vi "hardware_initialize_hardware.vi"(8 "error in (no error)":errorcluster, 11 "thorlabs_kinesis in":refnum<class "thorlabs_kinesis.lvclass">) -> (0 "error out":errorcluster, 3 "thorlabs_kinesis out":refnum<class "thorlabs_kinesis.lvclass">)   [LabVIEW 2015, in "thorlabs_kinesis.lvclass"]
uses:
  thorlabs_kinesis.lvclass
  thorlabs_kinesis.lvclass/thorlabs_kinesis.ctl
  thorlabs_drivers/Thorlabs.MotionControl.Benchtop.Piezo.dll
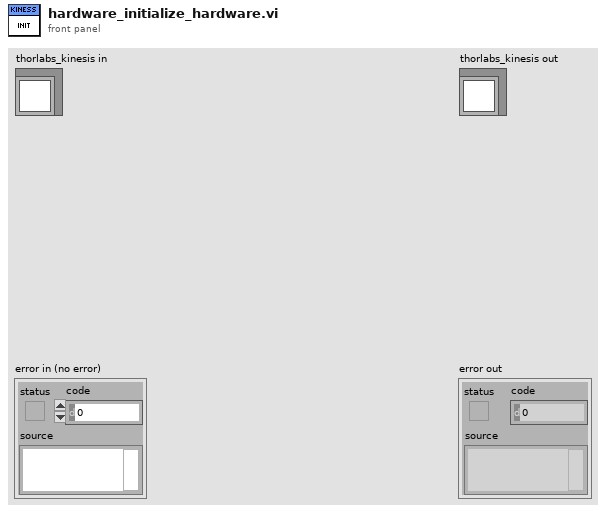
[diagram p1: front panel]
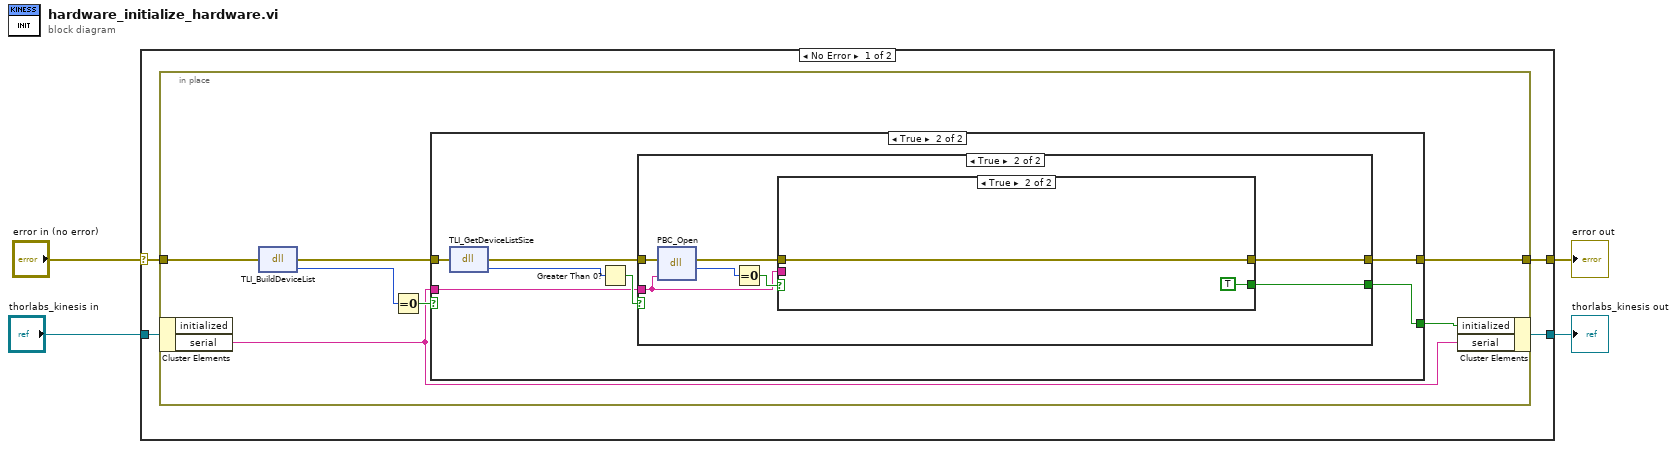
[diagram p0: block diagram]
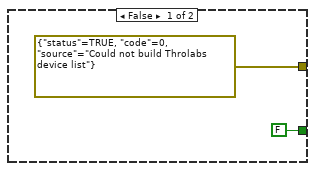
[diagram p2: hidden frame]
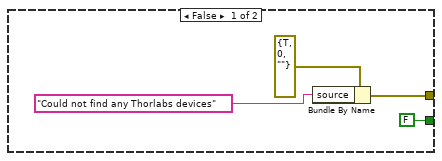
[diagram p3: hidden frame]
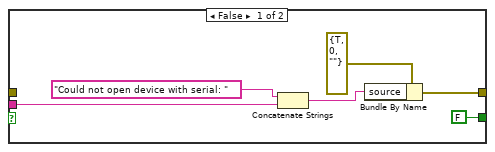
[diagram p4: hidden frame]
diagram:
  n1 = case shown="No Error" "error in (no error)" {
    selector: "error in (no error)" -> [w7 w44]
    tunnel: "thorlabs_kinesis in" -> [w8 w45]
    tunnel: [w6 w44] -> w2
    tunnel: [w5 w45] -> w1
    frame No Error {
      n2 = in-place {
        in-place-border: w7 -> [w15]
        in-place-border: [w10] -> w6
        n3 = in-place-cluster #1(w8) -> ("serial"=w11:string)  [unwired: 1 out]
        n4 = dll-call lib="C:/Users/bspoka/Documents/LabVIEW Data/lview_180307/Stage Class/Thorlabs Kinesis/thorlabs_drivers/Thorlabs.MotionControl.Benchtop.Piezo.dll" fn="TLI_BuildDeviceList"(error in=w15) -> (error out=w12:errorcluster, "return type"=w14:i16)  [unwired: 2 in, 1 out]
        n5 = Equal To 0?(x=w14) -> (x = 0?=w13:bool)
        n6 = case shown="True" w13 {
          tunnel: w12 -> [_ w24]
          tunnel: w11 -> [_ w20]
          tunnel: [errorcluster {"status"=TRUE, "code"=0, "source"="Could not build Throlabs device list"} ("error out") w19] -> w10
          tunnel: [FALSE w18] -> w9
          frame False {
          }
          frame True {
            n7 = dll-call lib="C:/Users/bspoka/Documents/LabVIEW Data/lview_180307/Stage Class/Thorlabs Kinesis/thorlabs_drivers/Thorlabs.MotionControl.Benchtop.Piezo.dll" fn="TLI_GetDeviceListSize"(error in=w24) -> (error out=w21:errorcluster, "return type"=w23:i16)  [unwired: 2 in, 1 out]
            n8 = Greater Than 0?(x=w23) -> (x > 0?=w22:bool)
            n9 = case shown="True" w22 {
              tunnel: w21 -> [_ w35]
              tunnel: w20 -> [_ w30]
              tunnel: [w27 w31] -> w19
              tunnel: [FALSE w29] -> w18
              frame False {
                n10 = Bundle By Name(cluster=errorcluster {"status"=TRUE, "code"=0, "source"=""} ("error out"), "source"="Could not find any Thorlabs devices") -> (w27:errorcluster)
              }
              frame True {
                n11 = dll-call lib="C:/Users/bspoka/Documents/LabVIEW Data/lview_180307/Stage Class/Thorlabs Kinesis/thorlabs_drivers/Thorlabs.MotionControl.Benchtop.Piezo.dll" fn="PBC_Open"(error in=w35, "serial"=w30) -> (error out=w32:errorcluster, "return type"=w34:i16)  [unwired: 3 in, 1 out]
                n12 = Equal To 0?(x=w34) -> (x = 0?=w33:bool)
                n13 = case shown="True" w33 {
                  tunnel: w32 -> [_ w43]
                  tunnel: [w37 w43] -> w31
                  tunnel: w30 -> [w39 _]
                  tunnel: [FALSE TRUE] -> w29
                  frame False {
                    n14 = Concatenate Strings("Could not open device with serial: " ("source"), w39) -> (w38:string)
                    n15 = Bundle By Name(cluster=errorcluster {"status"=TRUE, "code"=0, "source"=""} ("error out"), "source"=w38) -> (w37:errorcluster)
                  }
                  frame True {
                  }
                }
              }
            }
          }
        }
        n16 = in-place-cluster #1("initialized"=w9, "serial"=w11) -> (w5:refnum<class "thorlabs_kinesis.lvclass">)
      }
    }
    frame Error {
    }
  }
  "error out" <- w2
  "thorlabs_kinesis out" <- w1
